vi "Clear.vi"(8 "error in (no error)":errorcluster, 11 "Report Generator In":refnum<class "Result Collector.lvclass">) -> (0 "error out":errorcluster, 3 "Report Generator Out":refnum<class "Result Collector.lvclass">)   [LabVIEW 2020, in "Result Collector.lvclass"]
uses:
  Result Collector.lvclass
  Result Collector.lvclass/Result Collector.ctl
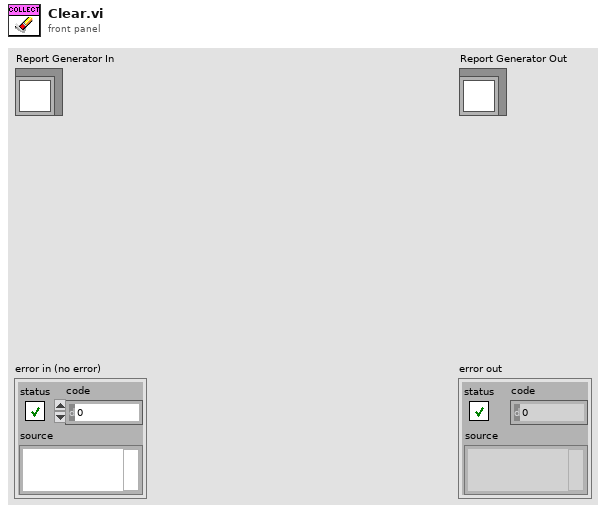
[diagram p1: front panel]
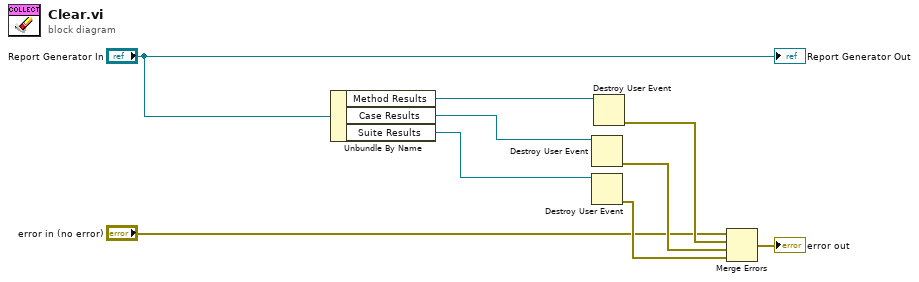
[diagram p0: block diagram]
diagram:
  n1 = Unbundle By Name("Report Generator In") -> ("Method Results"=w7:refnum<user-event>, "Case Results"=w6:refnum<user-event>, "Suite Results"=w5:refnum<user-event>)
  n2 = Destroy User Event(user event=w6) -> (error out=w3:errorcluster)  [unwired: 1 in]
  n3 = Destroy User Event(user event=w5) -> (error out=w2:errorcluster)  [unwired: 1 in]
  n4 = Destroy User Event(user event=w7) -> (error out=w4:errorcluster)  [unwired: 1 in]
  n5 = Merge Errors("error in (no error)", w4, w3, w2) -> (→"error out":errorcluster)
  "Report Generator Out" <- "Report Generator In"
